vi "EnumerateMethods.vi"(8 "error in (no error)":errorcluster, 11 "Web Service Importer in":refnum<k24>) -> (0 "error out":errorcluster, 1 "ServiceName":string, 2 "Methods":string[](array[string]), 3 "Web Service Importer out":refnum<k24>, 5 "MethodsHelp":string[](array[string]))   [LabVIEW 2017]
uses:
  e:/builds/penguin/labview/branches/2017/dev/dist/resource/WebServiceUtils.dll
  resource/WebServiceUtils.dll
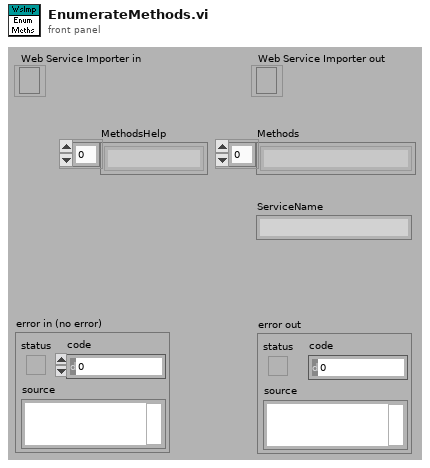
[diagram p1: front panel]
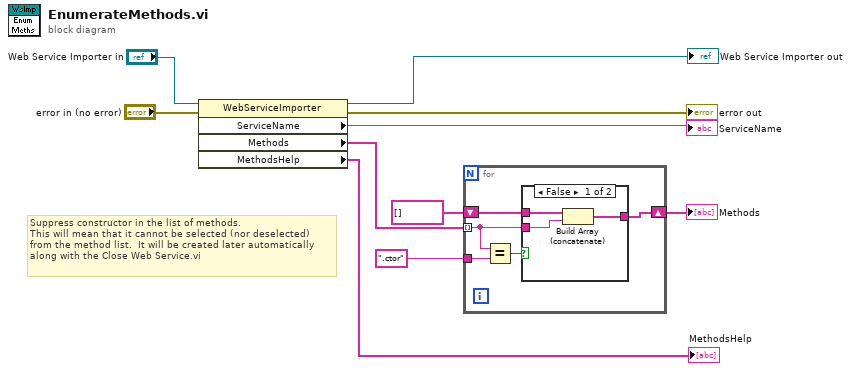
[diagram p0: block diagram]
diagram:
  # "Suppress constructor in the list of methods.\nThis will mean that it cannot be selected (nor deselected)\nfrom the method list.  It will be created later automatically\nalong with the Close Web Service.vi"
  n1 = property class="WebServiceImporter"(reference="Web Service Importer in", error in="error in (no error)") -> (reference out=→"Web Service Importer out":refnum<k24>, error out=→"error out":errorcluster, "ServiceName"=→"ServiceName":string, "Methods"=w3:string[], "MethodsHelp"=→"MethodsHelp":string[])
  n2 = for {
    tunnel: w3 -> [w11] mode=indexing
    tunnel: ".ctor" -> [w15]
    shift-right: [w13] -> w2
    shift-left: string[] [] -> [w12]
    n3 = Equal?(x=w11, y=w15) -> (x = y?=w14:bool)
    n4 = case shown="False" w14 {
      tunnel: [w18 w19] -> w13
      tunnel: w12 -> [w17 w19]
      tunnel: w11 -> [w16 _]
      frame False {
        n5 = Build Array (concatenate)(w17, w16) -> (w18:string[])
      }
      frame True {
      }
    }
  }
  "Methods" <- w2
